vi "LIA Simulation Sine Cosine Host.vi"() -> ()   [LabVIEW 2017]
uses:
  <vilib>/rvi/FXPMathLib/FxpSinAndCos/subVIs/nifxpmath_SinAndCos_SimConfig.ctl
  <vilib>/Analysis/2dsp.llb/Complex FFT.vi
  <vilib>/rvi/FXPMathLib/FxpSinAndCos/simVIs/DllFxpSinAndCosTemp_sub.vi
  <vilib>/rvi/FXPMathLib/FxpAdd/XNode/nifxpmath_Add.xnode
  <vilib>/rvi/FXPMathLib/FxpSinAndCos/XNode/nifxpmath_SinAndCos.xnode
  <vilib>/Analysis/NI_AALPro.lvlib
  <vilib>/rvi/FXPMathLib/sim/FxpSim.dll
  <vilib>/rvi/FXPMathLib/FxpMul/XNode/nifxpmath_Multiplier.xnode
  <vilib>/rvi/FXPMathLib/FxpSub/XNode/nifxpmath_Sub.xnode
  <vilib>/ptbypt/NI_PtbyPt.lvlib
  <vilib>/Analysis/NI_AALBase.lvlib
panel:
  out "Numeric Control 2":dbl
  out "Numeric Control  1":dbl
  out "standard deviation":dbl format="%0.2f"
  out "mean":dbl format="%0.2f"
  out "phase delta (pi rad) 2":fxp<+/-,25,1>
  out "Waveform Graph 2":cluster{"f0":dbl, "df":dbl, "magnitude":dbl[]}[](graph)
  in  "Frequency (Hz)":dbl=1000000.0 format="%#_p"
  in  "Sampling Rate (Hz)":dbl=100000000.0 format="%#_p"
  out "Waveform Graph":dbl[][](graph)
  out "phase delta (pi rad) 1":fxp<+/-,25,1>
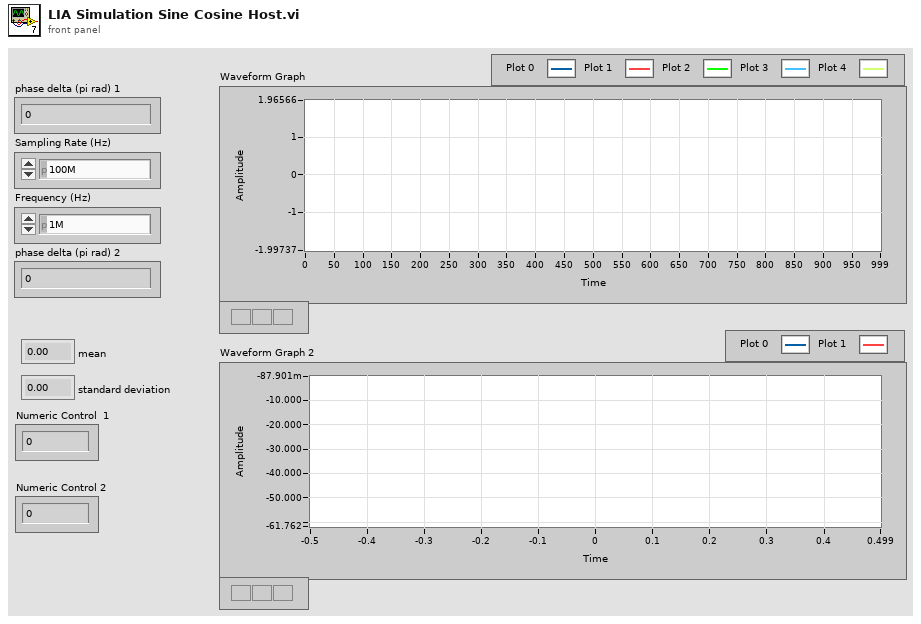
[diagram p1: front panel]
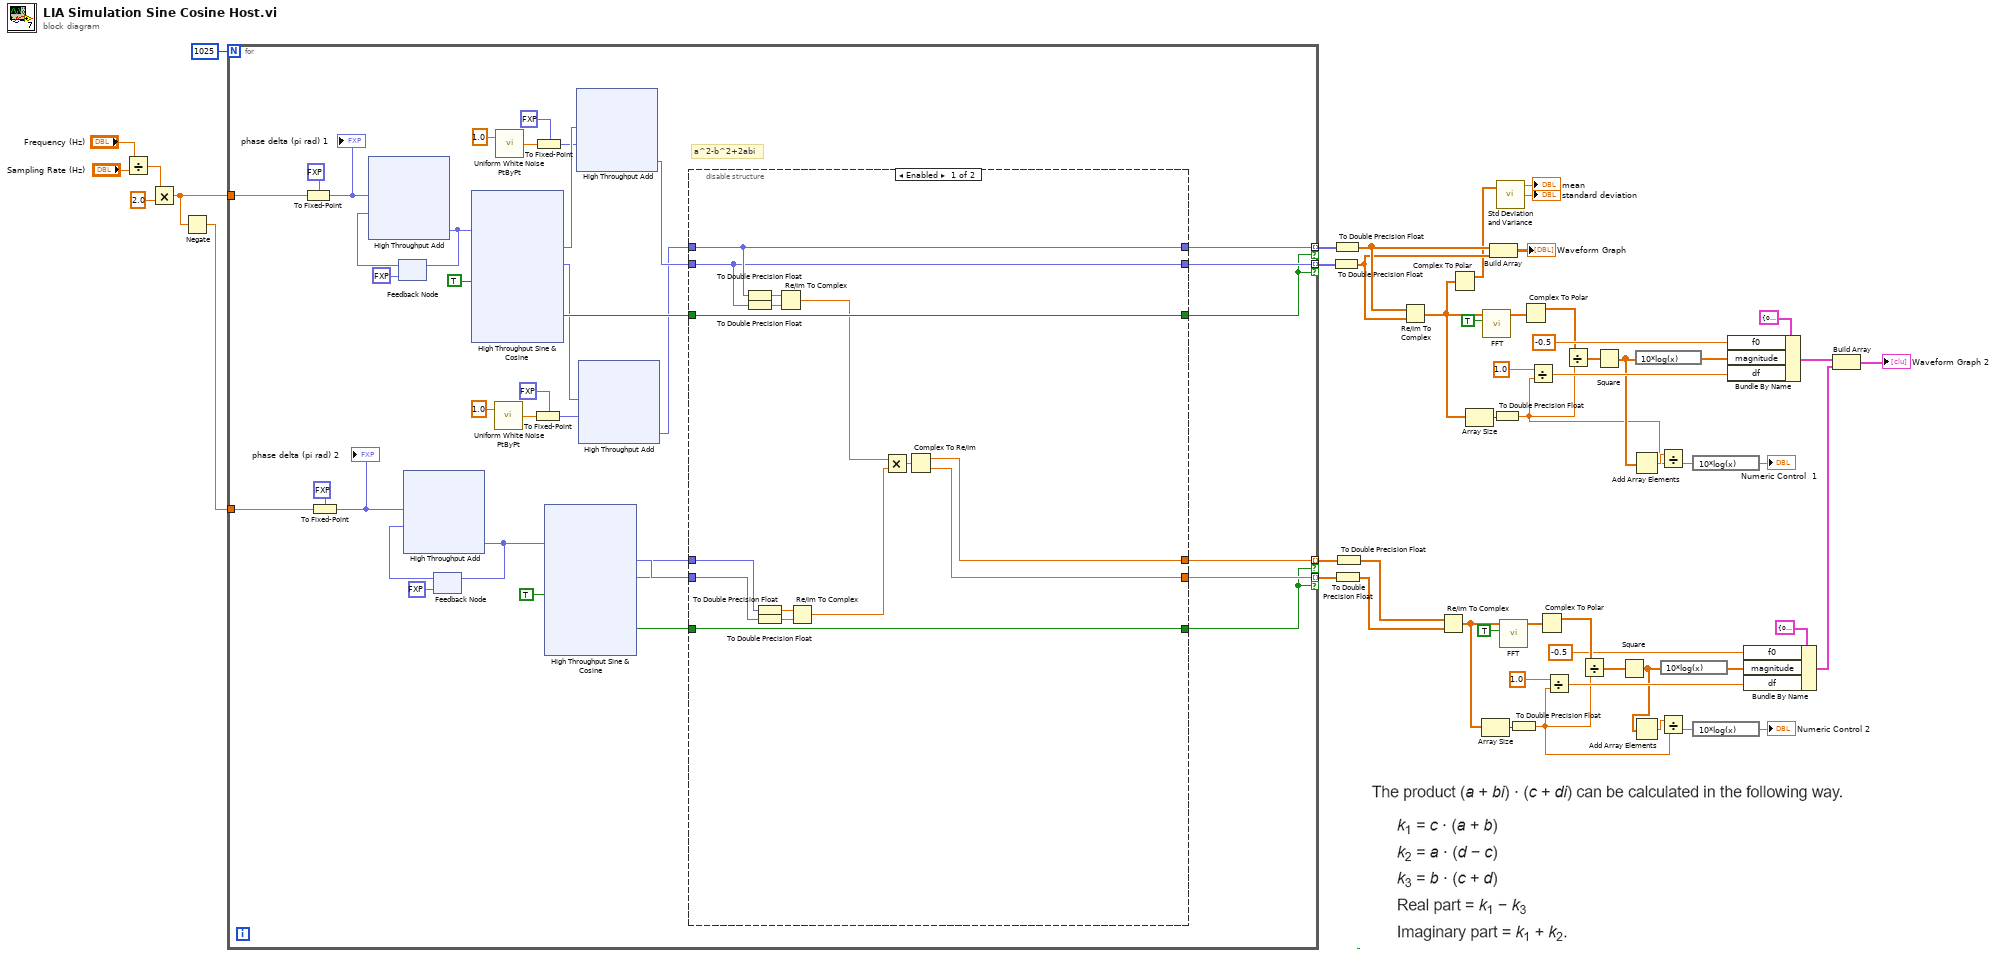
[diagram p0: block diagram]
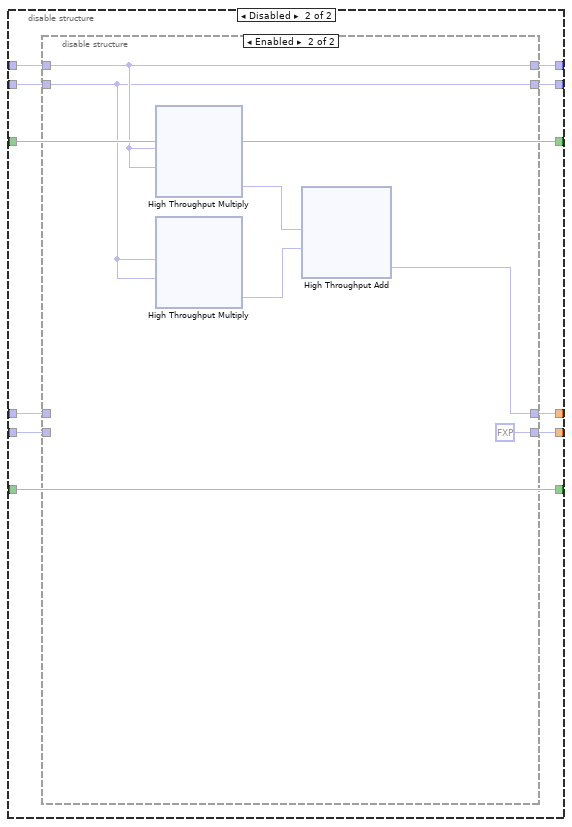
[diagram p2: hidden frame]
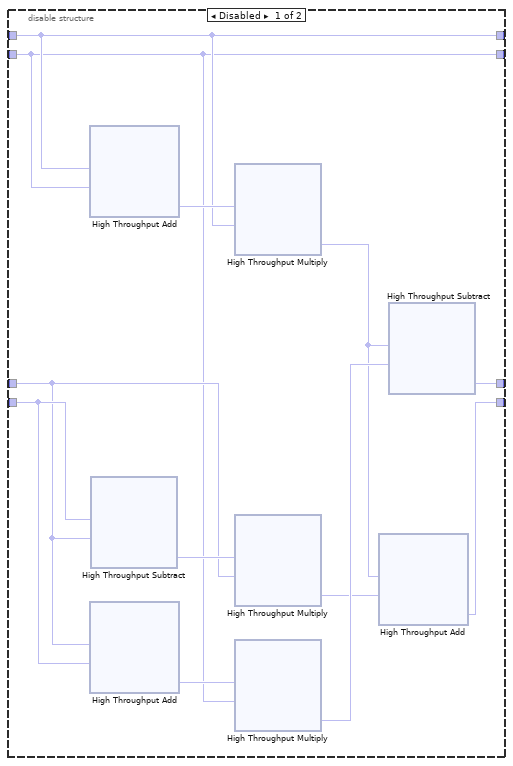
[diagram p3: hidden frame]
diagram:
  n1 = Divide(x="Frequency (Hz)", y="Sampling Rate (Hz)") -> (x/y=w51:dbl)
  n2 = Multiply(x=w51, y=2.0) -> (x*y=w16:dbl)
  n3 = Negate(x=w16) -> (-x=w15:dbl)
  n4 = for {
    N: 1025 -> [_]
    tunnel: [w75] -> w49 mode=indexing if=w71
    tunnel: w16 -> [w89]
    tunnel: [w74] -> w47 mode=indexing if=w71
    tunnel: [w85] -> w34 mode=indexing if=w73
    tunnel: [w84] -> w33 mode=indexing if=w73
    tunnel: w15 -> [w78]
    # "a^2-b^2+2abi"
    n5 = To Fixed-Point(fixed-point type=fxp<+/-,25,1> 0.0, number=w89) -> (fixed-point=w88:fxp<+/-,25,1>)
    "phase delta (pi rad) 1" <- w88
    n6 = To Fixed-Point(fixed-point type=fxp<+/-,25,1> 0.0 ("phase delta (pi rad)"), number=w78) -> (fixed-point=w81:fxp<+/-,25,1>)
    "phase delta (pi rad) 2" <- w81
    n7 = feedback #1(fxp<+/-,25,2> 0.0 ("x+y")) -> (w86:fxp<+/-,25,2>)
    n8 = xnode ("High Throughput Add")("x"=w88, "y"=w86) -> ("x+y"=w90:fxp<+/-,25,2>)
    n9 = feedback-in #1(w90) -> ()
    n10 = feedback #2(fxp<+/-,25,2> 0.0 ("x+y")) -> (w83:fxp<+/-,25,2>)
    n11 = xnode ("High Throughput Add")("x"=w81, "y"=w83) -> ("x+y"=w79:fxp<+/-,25,2>)
    n12 = feedback-in #2(w79) -> ()
    n13 = xnode "High Throughput Sine & Cosine"("x (pi)"=w90, "input valid"=TRUE) -> ("sin(x)"=w66:fxp<+/-,25,2>, "cos(x)"=w64:fxp<+/-,25,2>, "output valid"=w70:bool)  [unwired: 1 in, 1 out]
    n14 = call <vilib>:"Uniform White Noise PtByPt.vi"("amplitude"=1.0) -> ("uniform white noise"=w57:dbl)  [unwired: 2 in]
    n15 = call <vilib>:"Uniform White Noise PtByPt.vi"("amplitude"=1.0) -> ("uniform white noise"=w62:dbl)  [unwired: 2 in]
    n16 = To Fixed-Point(fixed-point type=fxp<+/-,25,1> 0.0, number=w57) -> (fixed-point=w55:fxp<+/-,25,1>)
    n17 = To Fixed-Point(fixed-point type=fxp<+/-,25,1> 0.0, number=w62) -> (fixed-point=w61:fxp<+/-,25,1>)
    n18 = xnode "High Throughput Sine & Cosine"("x (pi)"=w79, "input valid"=TRUE) -> ("sin(x)"=w77:fxp<+/-,25,2>, "cos(x)"=w76:fxp<+/-,25,2>, "output valid"=w72:bool)  [unwired: 1 in, 1 out]
    n19 = xnode ("High Throughput Add")("x"=w66, "y"=w61) -> ("x+y"=w65:fxp<+/-,25,2>)
    n20 = xnode ("High Throughput Add")("x"=w64, "y"=w55) -> ("x+y"=w63:fxp<+/-,25,2>)
    n21 = disable-structure shown="Enabled" {
      disable-tunnel: [w99 w111] -> w85
      disable-tunnel: [w98 w110] -> w84
      disable-tunnel: w77 -> [w93 w109]
      disable-tunnel: w76 -> [w94 w108]
      disable-tunnel: [w96 w107] -> w75
      disable-tunnel: w65 -> [w95 w112]
      disable-tunnel: [w95 w106] -> w74
      disable-tunnel: w63 -> [w96 w113]
      disable-tunnel: [w101 w115] -> w73
      disable-tunnel: w72 -> [w101 w115]
      disable-tunnel: [w97 w114] -> w71
      disable-tunnel: w70 -> [w97 w114]
      frame Enabled {
        n22 = To Double Precision Float(number=w96) -> (double precision float=w104:dbl)
        n23 = To Double Precision Float(number=w95) -> (double precision float=w105:dbl)
        n24 = To Double Precision Float(number=w94) -> (double precision float=w103:dbl)
        n25 = To Double Precision Float(number=w93) -> (double precision float=w102:dbl)
        n26 = Re/Im To Complex(1:w105, 2:w104) -> (0:w92:cdb)
        n27 = Re/Im To Complex(1:w102, 2:w103) -> (0:w91:cdb)
        n28 = Multiply(x=w92, y=w91) -> (x*y=w100:cdb)
        n29 = Complex To Re/Im(x + iy=w100) -> (x=w99:dbl, y=w98:dbl)
      }
      frame Disabled {
        n30 = disable-structure shown="Enabled" {
          disable-tunnel: w113 -> [w117 w131]
          disable-tunnel: w112 -> [w116 w130]
          disable-tunnel: [w123 w128] -> w111
          disable-tunnel: [w120 fxp<+/-,21,3> 0.0 ("x-y")] -> w110
          disable-tunnel: w109 -> [w119 _]
          disable-tunnel: w108 -> [w118 _]
          disable-tunnel: [w117 w131] -> w107
          disable-tunnel: [w116 w130] -> w106
          frame Disabled {
            n31 = xnode ("High Throughput Add")("x"=w117, "y"=w116) -> ("x+y"=w127:fxp<+/-,22,2>)
            n32 = xnode ("High Throughput Add")("x"=w118, "y"=w119) -> ("x+y"=w125:fxp<+/-,22,2>)
            n33 = xnode ("High Throughput Subtract")("x"=w119, "y"=w118) -> ("x-y"=w126:fxp<+/-,26,3>)
            n34 = xnode ("High Throughput Multiply")("x"=w127, "y"=w117) -> ("x*y"=w122:fxp<+/-,20,2>)
            n35 = xnode ("High Throughput Multiply")("x"=w126, "y"=w118) -> ("x*y"=w121:fxp<+/-,20,2>)
            n36 = xnode ("High Throughput Multiply")("x"=w125, "y"=w116) -> ("x*y"=w124:fxp<+/-,20,2>)
            n37 = xnode ("High Throughput Add")("x"=w122, "y"=w121) -> ("x+y"=w120:fxp<+/-,22,2>)
            n38 = xnode ("High Throughput Subtract")("x"=w122, "y"=w124) -> ("x-y"=w123:fxp<+/-,21,3>)
          }
          frame Enabled {
            n39 = xnode ("High Throughput Multiply")("x"=w131, "y"=w131) -> ("x*y"=w133:fxp<+/-,25,2>)
            n40 = xnode ("High Throughput Multiply")("x"=w130, "y"=w130) -> ("x*y"=w132:fxp<+/-,25,2>)
            n41 = xnode ("High Throughput Add")("x"=w133, "y"=w132) -> ("x+y"=w128:fxp<+/-,25,2>)
          }
        }
      }
    }
  }
  n42 = To Double Precision Float(number=w47) -> (double precision float=w45:dbl[])
  n43 = To Double Precision Float(number=w49) -> (double precision float=w46:dbl[])
  n44 = To Double Precision Float(number=w33) -> (double precision float=w17:dbl[])
  n45 = To Double Precision Float(number=w34) -> (double precision float=w18:dbl[])
  n46 = Re/Im To Complex(1:w45, 2:w46) -> (0:w14:cdb[])
  n47 = Re/Im To Complex(1:w17, 2:w18) -> (0:w31:cdb[])
  n48 = Complex To Polar(r * e^(i*theta)=w14) -> (r=w13:dbl[])  [unwired: 1 out]
  n49 = Array Size(array=w14) -> (size(s)=w35:i32)
  n50 = Array Size(array=w31) -> (size(s)=w32:i32)
  n51 = call-poly <vilib>:"FFT.vi"("shift?"=TRUE, "X"=w14) -> ("FFT {X}"=w48:cdb[])  [unwired: 8 in, 1 out]
  n52 = Build Array(w46, w45) -> (→"Waveform Graph":dbl[][])
  n53 = To Double Precision Float(number=w35) -> (double precision float=w7:dbl)
  n54 = call <vilib>:"Std Deviation and Variance.vi"("X"=w13) -> ("mean"=→"mean":dbl, "standard deviation"=→"standard deviation":dbl)  [unwired: 1 in, 1 out]
  n55 = call-poly <vilib>:"FFT.vi"("shift?"=TRUE, "X"=w31) -> ("FFT {X}"=w24:cdb[])  [unwired: 8 in, 1 out]
  n56 = To Double Precision Float(number=w32) -> (double precision float=w1:dbl)
  n57 = Complex To Polar(r * e^(i*theta)=w48) -> (r=w40:dbl[])  [unwired: 1 out]
  n58 = Divide(x=1.0 ("df"), y=w7) -> (x/y=w37:dbl)
  n59 = Complex To Polar(r * e^(i*theta)=w24) -> (r=w28:dbl[])  [unwired: 1 out]
  n60 = Divide(x=1.0 ("df"), y=w1) -> (x/y=w30:dbl)
  n61 = Divide(x=w40, y=w7) -> (x/y=w36:dbl[])
  n62 = Divide(x=w28, y=w1) -> (x/y=w20:dbl[])
  n63 = Square(x=w36) -> (x^2=w10:dbl[])
  n64 = Square(x=w20) -> (x^2=w2:dbl[])
  n65 = Add Array Elements(numeric array=w10) -> (sum=w9:dbl)
  n66 = Add Array Elements(numeric array=w2) -> (sum=w3:dbl)
  n67 = expression code="10*log(x)"(w10) -> (w21:dbl[])
  n68 = Divide(x=w9, y=w7) -> (x/y=w8:dbl)
  n69 = Divide(x=w3, y=w1) -> (x/y=w4:dbl)
  n70 = expression code="10*log(x)"(w2) -> (w19:dbl[])
  n71 = expression code="10*log(x)"(w8) -> (→"Numeric Control  1":dbl)
  n72 = expression code="10*log(x)"(w4) -> (→"Numeric Control 2":dbl)
  n73 = Bundle By Name(cluster=cluster{"f0":dbl, "df":dbl, "magnitude":dbl[]} {"f0"=0.0, "df"=0.0, "magnitude"=[]} ("Power Spectrum / PSD"), "f0"=-0.5, "magnitude"=w21, "df"=w37) -> (w38:cluster{"f0":dbl, "df":dbl, "magnitude":dbl[]})
  n74 = Bundle By Name(cluster=cluster{"f0":dbl, "df":dbl, "magnitude":dbl[]} {"f0"=0.0, "df"=0.0, "magnitude"=[]} ("Power Spectrum / PSD"), "f0"=-0.5, "magnitude"=w19, "df"=w30) -> (w22:cluster{"f0":dbl, "df":dbl, "magnitude":dbl[]})
  n75 = Build Array(w38, w22) -> (→"Waveform Graph 2":cluster{"f0":dbl, "df":dbl, "magnitude":dbl[]}[])
